vi "Process New Connection.vi"(8 "error in (no error)":errorcluster, 10 "Connection Reference":refnum<data-value>, 11 "PersistantConnectionHandler in":refnum<class "PersistantConnectionHandler.lvclass">) -> (0 "error out":errorcluster, 3 "PersistantConnectionHandler out":refnum<class "PersistantConnectionHandler.lvclass">)   [LabVIEW 2019, in "PersitantConnectionHandler.lvlib" / "PersistantConnectionHandler.lvclass"]
uses:
  <vilib>/gpm_packages/@cs/Network-interface/Source/PersistantConnectionHandler/PersistantConnectionHandler/PersistantConnectionHandler.lvclass
  C:/Program Files/National Instruments/LabVIEW 2019/vi.lib/gpm_packages/@cs/Network-interface/Source/Logged Actor/LoggedActor.lvclass
  C:/Program Files/National Instruments/LabVIEW 2019/vi.lib/ActorFramework/Actor/Actor.lvclass
  <vilib>/gpm_packages/@cs/Network-interface/Source/Connection Reference/Connection Reference/Connection Reference.lvclass
  <vilib>/gpm_packages/@cs/event-logger/Source/Composed Log/Types/Log Level.ctl
  <vilib>/gpm_packages/@cs/Network-interface/Source/Logged Actor/LoggedActor.lvclass/LoggedActor.ctl
  <vilib>/gpm_packages/@cs/Network-interface/Source/PersistantConnectionHandler/PersistantConnectionHandler/PersistantConnectionHandler.lvclass/PersistantConnectionHandler.ctl
  <vilib>/gpm_packages/@cs/Network-interface/Source/ProtectedConnectionReader/ProtectedConnectionReader.lvclass/ProtectedConnectionReader.ctl
  <vilib>/gpm_packages/@cs/Network-interface/Source/ProtectedConnectionWriter/ProtectedConnectionWriter.lvclass/ProtectedConnectionWriter.ctl
  <vilib>/gpm_packages/@cs/Network-interface/Source/Connection Reference/Connection Reference/Connection Reference.lvclass/Connection Reference.ctl
  <vilib>/gpm_packages/@cs/event-logger/Source/Composed Log/LoggerReference/LoggerReference.lvclass/LoggerReference.ctl
  <vilib>/gpm_packages/@cs/event-logger/Source/Composed Log/LoggerReference/Log Event.vi
  <vilib>/gpm_packages/@cs/event-logger/Source/Composed Log/LoggerReference/Log.vi
  <vilib>/gpm_packages/@cs/event-logger/Source/Composed Log/LoggerReference/Get Valid Event Time.vi
  <vilib>/gpm_packages/@cs/event-logger/Source/Composed Log/LoggerReference/Remove Stale Logs.vi
  <vilib>/gpm_packages/@cs/Network-interface/Source/ConnectionManager/ConnectionManager/ConnectionManager.lvclass
  <vilib>/gpm_packages/@cs/Network-interface/Source/ProtectedConnectionReader/ProtectedConnectionReader.lvclass
  <vilib>/gpm_packages/@cs/Network-interface/Source/ProtectedConnectionWriter/ProtectedConnectionWriter.lvclass
  <vilib>/gpm_packages/@cs/Network-interface/Source/Connection Reference/IConnection/IConnection.lvclass
  <vilib>/gpm_packages/@cs/Network-interface/Source/MessagingInterfaces/IConnectionStateChangeCallback/IConnectionStateChangeCallback.lvclass
  <vilib>/ActorFramework/Actor/Actor.lvclass
  <vilib>/gpm_packages/@cs/Network-interface/Source/Logged Actor/LoggedActor.lvclass
  <vilib>/gpm_packages/@cs/event-logger/Source/Composed Log/Composed Log.lvlib
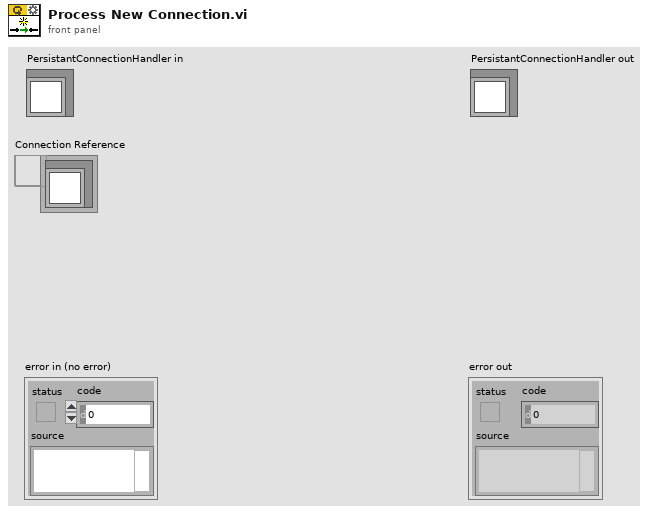
[diagram p1: front panel]
types:
  T1 = typedef "Composed Log.lvlib/Log Level.ctl" = enum16{"Debug", "Info", "Warning", "Error", "Critical"}
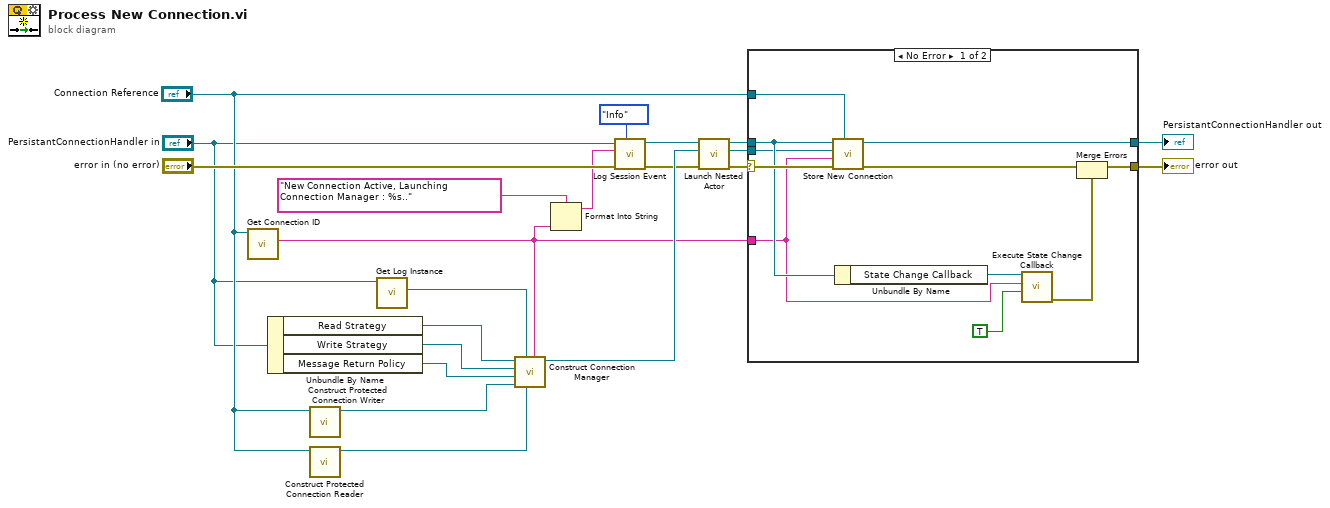
[diagram p0: block diagram]
diagram:
  n1 = call <vilib>:"Get Connection ID.vi"("Connection Reference In"="Connection Reference") -> ("ID"=w1:string)  [unwired: 8 in, 2 out]
  n2 = Unbundle By Name("PersistantConnectionHandler in") -> ("Read Strategy"=w17:refnum<class "IReadStrategy.lvclass">, "Write Strategy"=w16:refnum<class "IWriteStrategy.lvclass">, "Message Return Policy"=w12:refnum<class "IMessageReturnPolicy.lvclass">)
  n3 = call <vilib>:"Construct Protected Connection Writer.vi"("Connection Reference"="Connection Reference") -> ("ProtectedConnectionWriter out"=w15:refnum<class "ProtectedConnectionWriter.lvclass">)  [unwired: 10 in]
  n4 = call <vilib>:"Construct Protected Connection Reader.vi"("Connection Reference"="Connection Reference") -> ("ProtectedConnectionReader out"=w14:refnum<class "ProtectedConnectionReader.lvclass">)  [unwired: 10 in]
  n5 = call <vilib>:"Get Log Instance.vi"("LoggedActor in"="PersistantConnectionHandler in") -> ("Log Instance"=w13:refnum<class "LoggerReference.lvclass">)  [unwired: 8 in, 2 out]
  n6 = call <vilib>:"Construct Connection Manager.vi"("ID"=w1, "ProtectedConnectionReader"=w14, "Log Instance"=w13, "ProtectedConnectionWriter"=w15, "Message Return Policy"=w12, "Write Policy"=w16, "Read Policy"=w17) -> ("ConnectionManager out"=w18:refnum<class "ConnectionManager.lvclass">)  [unwired: 4 in]
  n7 = Format Into String(format string="New Connection Active, Launching Connection Manager : %s..", w1) -> (resulting string=w4:string)  [unwired: 2 in, 1 out]
  n8 = call <vilib>:"Log Session Event.vi"("Event Level"=Log_Level."Info", "error in (no error)"="error in (no error)", "Event Data"=w4, "SessionActor in"="PersistantConnectionHandler in") -> ("error out"=w7:errorcluster, "SessionActor out"=w9:refnum<class "PersistantConnectionHandler.lvclass">)  [unwired: 6 in]
  n9 = call <vilib>:"Launch Nested Actor.vi"("error in (no error)"=w7, "Nested Actor"=w18, "Caller Actor in"=w9) -> ("error out"=w11:errorcluster, "Nested Actor's Enqueuer"=w20:refnum<class "Message Enqueuer.lvclass">, "Caller Actor out"=w19:refnum<class "PersistantConnectionHandler.lvclass">)  [unwired: 6 in]
  n10 = case shown="No Error" w11 {
    selector: w11 -> [w28 w33]
    tunnel: [w26 w34] -> w21
    tunnel: w20 -> [w24 _]
    tunnel: w19 -> [w25 w34]
    tunnel: [w30 w33] -> w10
    tunnel: w1 -> [w23 _]
    tunnel: "Connection Reference" -> [w22 _]
    frame No Error {
      n11 = call-dynamic "Store New Connection.vi"("Connection Reference"=w22, "error in (no error)"=w28, "Active Connection ID"=w23, "Connection Manager Queue"=w24, "PersistantConnectionHandler in"=w25) -> ("error out"=w27:errorcluster, "PersistantConnectionHandler out"=w26:refnum<class "PersistantConnectionHandler.lvclass">)  [unwired: 5 in]
      n12 = Unbundle By Name(w25) -> ("State Change Callback"=w32:refnum<class "IConnectionStateChangeCallback.lvclass">)
      n13 = call-dynamic "Execute State Change Callback.vi"("Connection State"=TRUE, "Connection ID"=w23, "IConnectionStateChangeCallback in"=w32) -> ("error out"=w29:errorcluster)  [unwired: 8 in]
      n14 = Merge Errors(w27, w29) -> (w30:errorcluster)
    }
    frame Error {
    }
  }
  "error out" <- w10
  "PersistantConnectionHandler out" <- w21
